vi "AllTests.vi"(0 "VI in":refnum<vi>, 1 "Label":string, 11 "error in (no error)":errorcluster) -> (4 "VI out":refnum<vi>, 15 "error out":errorcluster)   [LabVIEW 2016, in "DronaTest.lvlib"]
uses:
  DronaTest.lvlib
  <vilib>/addons/_JKI Toolkits/Caraya/classes/Assert/Assert Not Error.vi
  <vilib>/addons/_JKI Toolkits/Caraya/classes/Assert/Assert.lvclass
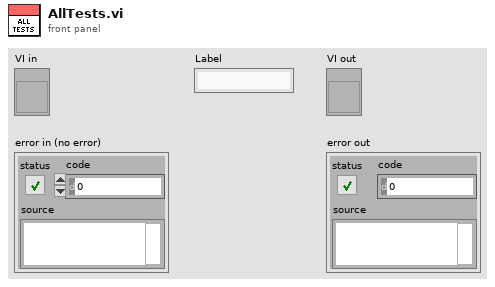
[diagram p1: front panel]
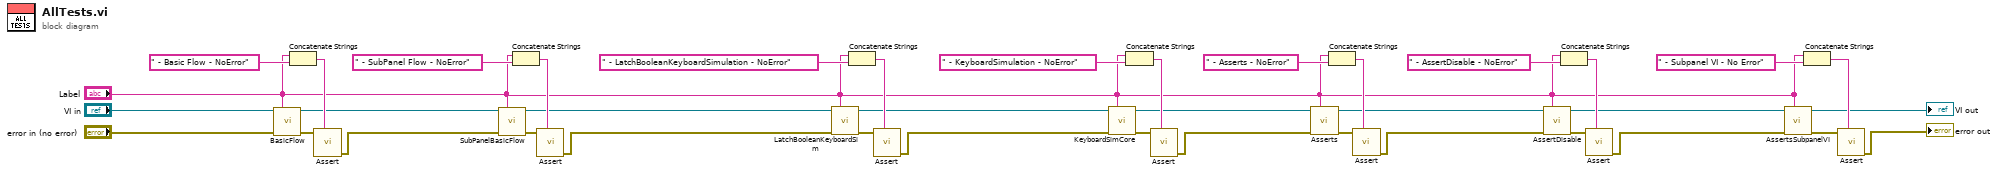
[diagram p0: block diagram]
diagram:
  n1 = call "BasicFlow.vi"("VI Reference In"="VI in", "Label (VI Title)"="Label", "error in (no error)"="error in (no error)") -> ("VI Reference Out"=w31:refnum<vi>, "error out"=w30:errorcluster)  [unwired: 11 in]
  n2 = Concatenate Strings("Label", " - Basic Flow - NoError" ("string")) -> (w32:string)
  n3 = call-poly <vilib>:"Assert.vi"("Label"=w32, "Not Error?"=w30) -> ("error out"=w29:errorcluster)  [unwired: 9 in]
  n4 = call "SubPanelBasicFlow.vi"("VI Reference In"=w31, "Label (VI Title)"="Label", "error in (no error)"=w29) -> ("VI Reference Out"=w21:refnum<vi>, "error out"=w26:errorcluster)  [unwired: 11 in]
  n5 = Concatenate Strings("Label", " - SubPanel Flow - NoError" ("string")) -> (w28:string)
  n6 = call-poly <vilib>:"Assert.vi"("Label"=w28, "Not Error?"=w26) -> ("error out"=w25:errorcluster)  [unwired: 9 in]
  n7 = call "LatchBooleanKeyboardSim.vi"("VI Reference In"=w21, "Label (VI Title)"="Label", "error in (no error)"=w25) -> ("VI Reference Out"=w18:refnum<vi>, "error out"=w22:errorcluster)  [unwired: 11 in]
  n8 = Concatenate Strings("Label", " - LatchBooleanKeyboardSimulation - NoError" ("string")) -> (w23:string)
  n9 = call-poly <vilib>:"Assert.vi"("Label"=w23, "Not Error?"=w22) -> ("error out"=w16:errorcluster)  [unwired: 9 in]
  n10 = call "KeyboardSimCore.vi"("VI Reference In"=w18, "Label (VI Title)"="Label", "error in (no error)"=w16) -> ("VI Reference Out"=w12:refnum<vi>, "error out"=w17:errorcluster)  [unwired: 11 in]
  n11 = Concatenate Strings("Label", " - KeyboardSimulation - NoError" ("string")) -> (w20:string)
  n12 = call-poly <vilib>:"Assert.vi"("Label"=w20, "Not Error?"=w17) -> ("error out"=w11:errorcluster)  [unwired: 9 in]
  n13 = call "Asserts.vi"("VI Reference In"=w12, "Label (VI Title)"="Label", "error in (no error)"=w11) -> ("VI Reference Out"=w8:refnum<vi>, "error out"=w15:errorcluster)  [unwired: 11 in]
  n14 = Concatenate Strings("Label", " - Asserts - NoError" ("string")) -> (w13:string)
  n15 = call-poly <vilib>:"Assert.vi"("Label"=w13, "Not Error?"=w15) -> ("error out"=w7:errorcluster)  [unwired: 9 in]
  n16 = call "AssertDisable.vi"("VI Reference In"=w8, "Label (VI Title)"="Label", "error in (no error)"=w7) -> ("VI Reference Out"=w5:refnum<vi>, "error out"=w6:errorcluster)  [unwired: 11 in]
  n17 = Concatenate Strings("Label", " - AssertDisable - NoError" ("string")) -> (w10:string)
  n18 = call-poly <vilib>:"Assert.vi"("Label"=w10, "Not Error?"=w6) -> ("error out"=w4:errorcluster)  [unwired: 9 in]
  n19 = call "AssertsSubpanelVI.vi"("VI Reference In"=w5, "Label (VI Title)"="Label", "error in"=w4) -> ("VI Reference Out"=→"VI out":refnum<vi>, "error out"=w3:errorcluster)  [unwired: 11 in]
  n20 = Concatenate Strings("Label", " - Subpanel VI - No Error" ("string")) -> (w34:string)
  n21 = call-poly <vilib>:"Assert.vi"("Label"=w34, "Not Error?"=w3) -> ("error out"=→"error out":errorcluster)  [unwired: 9 in]
